vi "Get - Registration Info.vi"(0 "reference in":refnum<class "Registration.lvclass">, 5 "error in (no error)":errorcluster) -> (13 "Registration Info":T1, 14 "reference out":refnum<class "Registration.lvclass">, 19 "error out":errorcluster)   [LabVIEW 2022 SP3, in "Registration.lvclass"]
uses:
  Registration.lvclass
  protected/Registration Info.ctl
  utils/Registration Type.ctl
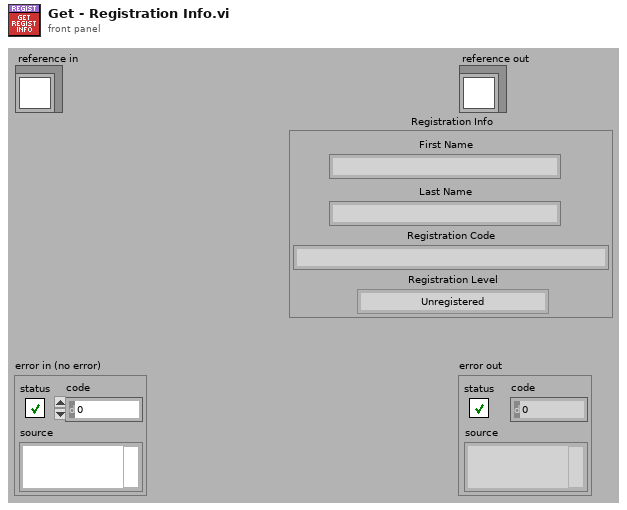
[diagram p1: front panel]
types:
  T1 = typedef "Registration.lvclass/Registration Info.ctl" = cluster{"First Name":string, "Last Name":string, "Registration Code":string, "Registration Level":T2}
  T2 = typedef "Registration.lvclass/Registration Type.ctl" = enum16{"Unregistered", "Registered - Full Activation", "Not Required- Full Activation"}
  T3 = typedef "Registration.lvclass/ObjectAttributes.ctl" = cluster{"Registration Info":T1, "Object Origin":enum16{"New/Created", "Existing"}}
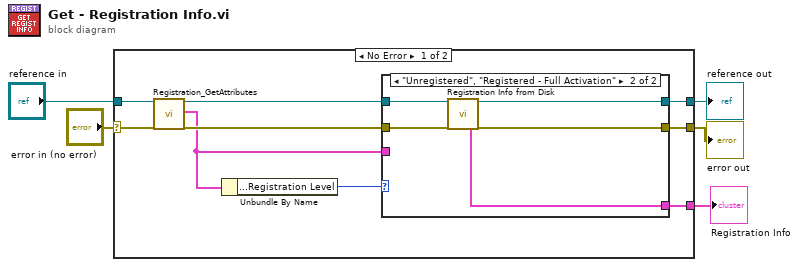
[diagram p0: block diagram]
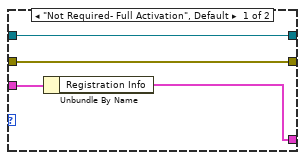
[diagram p2: hidden frame]
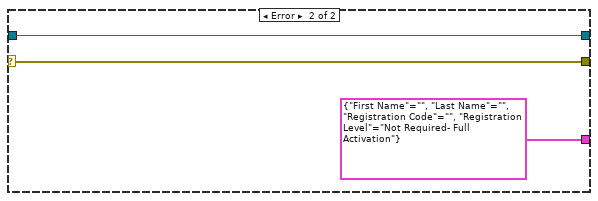
[diagram p3: hidden frame]
diagram:
  n1 = case shown="No Error" "error in (no error)" {
    selector: "error in (no error)" -> [w14 w26]
    tunnel: [w9 w26] -> w4
    tunnel: [w10 w25] -> w2
    tunnel: "reference in" -> [w13 w25]
    tunnel: [w7 T1 {"First Name"="", "Last Name"="", "Registration Code"="", "Registration Level"=enum."Not Required- Full Activation"} ("Registration Info")] -> w1
    frame No Error {
      n2 = call "Registration_GetAttributes.vi"("reference in"=w13, "error in (no error)"=w14) -> ("reference out"=w12:refnum<class "Registration.lvclass">, "attributes"=w6:T3, "error out"=w11:errorcluster)  [unwired: 14 in, 1 out]
      n3 = Unbundle By Name(w6) -> ("Registration Info.Registration Level"=w8:T2)
      n4 = case shown="\"Unregistered\", \"Registered - Full Activation\"" w8 {
        tunnel: w12 -> [w18 w23]
        tunnel: w11 -> [w17 w22]
        tunnel: [w18 w21] -> w10
        tunnel: [w17 w20] -> w9
        tunnel: [w15 w19] -> w7
        tunnel: w6 -> [w16 _]
        frame "Not Required- Full Activation", Default {
          n5 = Unbundle By Name(w16) -> ("Registration Info"=w15:T1)
        }
        frame "Unregistered", "Registered - Full Activation" {
          n6 = call "Registration Info from Disk.vi"("reference in"=w23, "error in (no error)"=w22) -> ("Registration Info"=w19:T1, "reference OUT"=w21:refnum<class "Registration.lvclass">, "error out"=w20:errorcluster)  [unwired: 15 in]
        }
      }
    }
    frame Error {
    }
  }
  "error out" <- w4
  "reference out" <- w2
  "Registration Info" <- w1
